vi "REMOVE SALE ITEM.vi"(11 "REFERENCES":T1) -> ()   [LabVIEW 2019]
uses:
  Controls/References Cluster.ctl
  <vilib>/userDefined/High Color/IMAQdx.ctl
  Controls/Custom Calendar/Custom Calendar.xctl
  <vilib>/addons/database/Connection.llb/DB Tools Open Connec (String).vi
  <vilib>/addons/database/_DB Variant To Data/Database Variant To Data.xnode
  <vilib>/addons/database/NI_Database_API.lvlib
types:
  T1 = typedef "References Cluster.ctl" = cluster{"MAIN PAGES":refnum<vi>, "ADD/EDIT ITEM REFERENCES":cluster{"Identifier":refnum<vi>, "BYU ICN #":refnum<vi>, "Item Description":refnum<vi>, "Comments":refnum<vi>, "Checked Out Date":refnum<vi>, "Due Date":refnum<vi>, "Check Out Location":refnum<vi>, "Reminder Count":refnum<vi>, "Most Recent Reminder Date":refnum<vi>, "BYU ID #":refnum<vi>, "Building/Room":refnum<vi>, "Location in Room":refnum<vi>, "Manual":refnum<vi>, "Manufacturer":refnum<vi>, "Model #":refnum<vi>, "Serial #":refnum<vi>, "Date Acquired":refnum<vi>, "ADD/EDIT ITEM LABEL":refnum<vi>, "ARCHIVE ITEM":refnum<vi>, "Archive Item Inputs":refnum<vi>, "Reminder Notes":refnum<vi>, "DUPLICATE ITEM":refnum<vi>}, "ADD/EDIT USER REFERENCES":cluster{"BYU ID # (##-###-####)":refnum<vi>, "First Name":refnum<vi>, "Last Name":refnum<vi>, "Phone Number (###-###-####)":refnum<vi>, "Email":refnum<vi>, "Department":refnum<vi>, "Graduation Status":refnum<vi>, "Anticipated Graduation Year":refnum<vi>, "Credit Score":refnum<vi>, "Date Added":refnum<vi>, "Graduation Clearance Date":refnum<vi>, "Picture File Name":refnum<vi>, "ADD/EDIT USER LABEL":refnum<vi>, "Department Map":refnum<vi>, "Status Map":refnum<vi>, "Anticipated Graduation Year Map":refnum<vi>, "User Agreement":refnum<vi>, "User Comments":refnum<vi>, "Camera":refnum<vi>}, "RETURN ITEM REFERENCES":cluster{"Item or Person:":refnum<vi>, "Search Return Results":refnum<vi>, "What are you searching for?":refnum<vi>}, "SEARCH DATABASE REFERENCES":cluster{"What to Search For:":refnum<vi>, "Where to Search":refnum<vi>, "Column to Search In":refnum<vi>, "Column to Sort By":refnum<vi>, "Search Database Results":refnum<vi>, "Inventory Column Selector":refnum<vi>, "User Column Selector":refnum<vi>, "Inventory Archive Column Selector":refnum<vi>, "User Archive Column Selector":refnum<vi>, "Sales Tracking Column Selector":refnum<vi>, "Checked In Archive Column Selector":refnum<vi>, "Restore User":refnum<vi>, "Date Range":refnum<vi>, "Dates Less Than":refnum<vi>, "Dates Greater Than":refnum<vi>, "Search Print Receipt":refnum<vi>, "Edit Sale Description":refnum<vi>}, "USER ITEMS REFERENCES":cluster{"USER'S INFORMATION":refnum<vi>, "User's Checked Out Items":refnum<vi>, "User Info Comments":refnum<vi>, "SEE USER INFO COMMENTS":refnum<vi>}, "EDIT ITEMS REFERENCES":cluster{"New Check Out Location":refnum<vi>, "Items to Edit":refnum<vi>, "Edit Items Due Date":refnum<vi>, "New Reminder Notes":refnum<vi>, "New Item Description":refnum<vi>}, "CHECK OUT ITEMS REFERENCES":cluster{"Enter Item:":refnum<vi>, "Check Out Items Due Date":refnum<vi>, "Check Out Location":refnum<vi>, "Items to be Checked Out":refnum<vi>, "Possible Items":refnum<vi>, "Altered Item Description":refnum<vi>}, "TRANSFER ITEMS REFERENCES":cluster{"Search Parameter":refnum<vi>, "What to Match":refnum<vi>, "Matching Individuals":refnum<vi>, "Items to be Transferred":refnum<vi>}, "SETTINGS REFERENCES":cluster{"PSC Database Settings":refnum<vi>, "PSC Sales Item Spreadsheet":refnum<vi>}, "PSC SALES REFERENCES":cluster{"BYU ID CARD #":refnum<vi>, "Sale Description":refnum<vi>, "Scan or Enter Item Name":refnum<vi>, "Items to be Sold":refnum<vi>, "Grand Total":refnum<vi>, "Item List":refnum<vi>}}
  T2 = cluster{"PSC Database Settings":refnum<vi>, "PSC Sales Item Spreadsheet":refnum<vi>}
  T3 = typedef "LVRowAndColumnTypeDef.ctl" = cluster{"Row":i32, "Column":i32}
  T4 = typedef "NI_Database_API.lvlib/Conn ObjectReference.ctl" = refnum<k1>
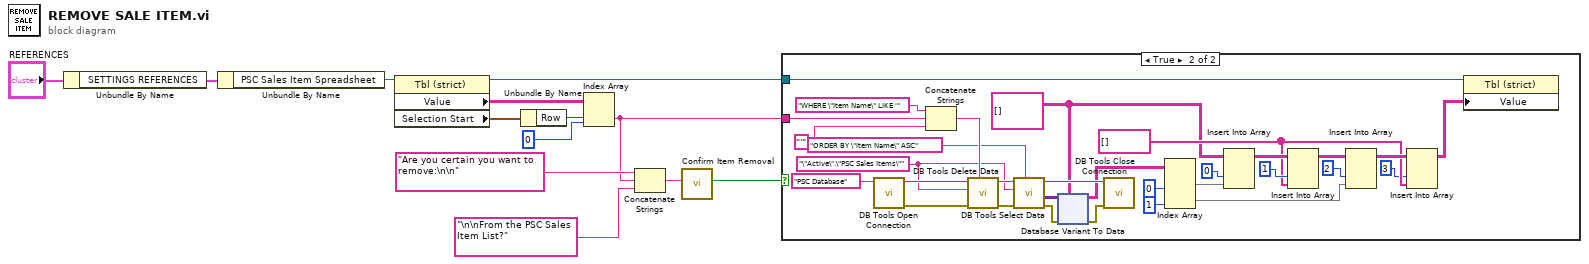
[diagram p0: block diagram]
diagram:
  n1 = Unbundle By Name("REFERENCES") -> ("SETTINGS REFERENCES"=w12:T2)
  n2 = Unbundle By Name(w12) -> ("PSC Sales Item Spreadsheet"=w11:refnum<vi>)
  n3 = property class="Tbl (strict)"(reference=w11) -> (reference out=w1:refnum<vi>, "Value"=w9:string[][], "Selection Start"=w10:T3)  [unwired: 1 in, 1 out]
  n4 = Unbundle By Name(w10) -> ("Row"=w8:i32)
  n5 = Index Array(array=w9, index (row)=w8, index (col)=0 ("disabled index (col)")) -> (element=w2:string)
  n6 = Concatenate Strings("Are you certain you want to remove:\n\n", w2, "\n\nFrom the PSC Sales Item List?") -> (w4:string)
  n7 = call "Confirm Item Removal"("Message"=w4) -> ("Yes, remove it"=w3:bool)  [unwired: 9 in, 1 out]
  n8 = case shown="True" w3 {
    tunnel: w2 -> [_ w41]
    tunnel: w1 -> [_ w14]
    frame False {
    }
    frame True {
      w19 = string[] []
      w16 = string[][] []
      w31 = "\"Active\".\"PSC Sales Items\""
      n9 = call-poly <vilib>:"DB Tools Open Connection.vi"("connection information"="PSC Database") -> ("error out"=w42:errorcluster, "connection reference"=w43:T4)  [unwired: 7 in]
      n10 = Concatenate Strings("WHERE \"Item Name\" LIKE '", w41, "'") -> (w38:string)
      n11 = call <vilib>:"DB Tools Delete Data.vi"("condition"=w38, "error in (no error)"=w42, "table"=w31, "connection reference"=w43) -> ("error out"=w32:errorcluster, "connection reference out"=w33:T4)  [unwired: 6 in]
      n12 = call <vilib>:"DB Tools Select Data.vi"("condition"="ORDER BY \"Item Name\" ASC", "error in (no error)"=w32, "table"=w31, "connection reference"=w33) -> ("error out"=w36:errorcluster, "data"=w37:variant[][], "connection reference out"=w35:T4)  [unwired: 2 in]
      n13 = xnode "Database Variant To Data"("database variant"=w37, "error in (no error)"=w36, "type"=w16) -> ("data"=w17:string[][], "error out"=w34:errorcluster)
      n14 = call <vilib>:"DB Tools Close Connection.vi"("error in (no error)"=w34, "connection reference"=w35) -> ()  [unwired: 5 in, 1 out]
      n15 = Index Array(array=w17, index (col) #1=0 ("disabled index (col)"), index (col) #2=1 ("index (col)")) -> (element #1=w25:string[], element #2=w21:string[])  [unwired: 2 in]
      n16 = Insert Into Array(array=w16, index (col)=0 ("disabled index (col)"), new element=w25) -> (w26:string[][])  [unwired: 1 in]
      n17 = Insert Into Array(array=w26, index (col)=1 ("disabled index (col)"), new element=w19) -> (w23:string[][])  [unwired: 1 in]
      n18 = Insert Into Array(array=w23, index (col)=2 ("disabled index (col)"), new element=w21) -> (w20:string[][])  [unwired: 1 in]
      n19 = Insert Into Array(array=w20, index (col)=3 ("disabled index (col)"), new element=w19) -> (w15:string[][])  [unwired: 1 in]
      n20 = property class="Tbl (strict)"(reference=w14, "Value"=w15) -> ()  [unwired: 1 in, 2 out]
    }
  }
